vi "Connect Terminals.vi"(7 "close source terminal refnum (T)":bool=TRUE, 8 "error in (no error)":errorcluster, 10 "sink terminal":refnum<vi>, 11 "source terminal":refnum<vi>) -> (0 "error out":errorcluster, 1 "connected?":bool)   [LabVIEW 2017, in "NI_Robotics_Scripting Utilities.lvlib"]
uses:
  <vilib>/robotics/Utilities/Scripting/NI_Robotics_Scripting Utilities.lvlib
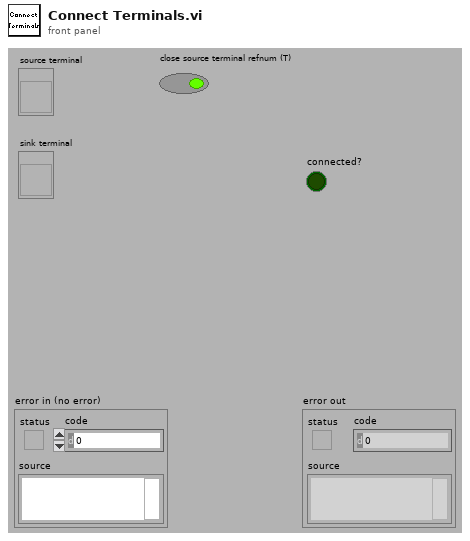
[diagram p1: front panel]
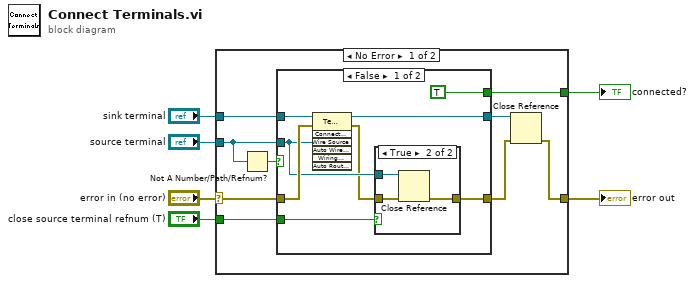
[diagram p0: block diagram]
diagram:
  n1 = case shown="No Error" "error in (no error)" {
    selector: "error in (no error)" -> [w8 w30]
    tunnel: "source terminal" -> [w14 _]
    tunnel: "sink terminal" -> [w13 _]
    tunnel: "close source terminal refnum (T)" -> [w12 _]
    tunnel: [w10 w30] -> w3
    tunnel: [w7 _] -> w1
    frame No Error {
      n2 = Not A Number/Path/Refnum?(number/path/refnum=w14) -> (NaN/Path/Refnum?=w15:bool)
      n3 = case shown="False" w15 {
        tunnel: w14 -> [w20 _]
        tunnel: w13 -> [w23 w28]
        tunnel: w8 -> [w22 w29]
        tunnel: [w19 w29] -> w9
        tunnel: w12 -> [w21 _]
        tunnel: [w17 w28] -> w11
        tunnel: [TRUE _] -> w7
        frame False {
          n4 = invoke class="Term" method="Connect Wire"(reference=w23, error in=w22, "Wire Source"=w20) -> (reference out=w17:refnum<vi>, error out=w18:errorcluster)  [unwired: 4 in, 5 out]
          n5 = case shown="True" w21 {
            tunnel: w20 -> [_ w27]
            tunnel: w18 -> [w24 w26]
            tunnel: [w24 w25] -> w19
            frame False {
            }
            frame True {
              n6 = Close Reference(reference=w27, error in (no error)=w26) -> (error out=w25:errorcluster)
            }
          }
        }
        frame True {
        }
      }
      n7 = Close Reference(reference=w11, error in (no error)=w9) -> (error out=w10:errorcluster)
    }
    frame Error {
    }
  }
  "error out" <- w3
  "connected?" <- w1
